vi "Check If Winner Board.vi"(9 "Matriz Status In":bool[][](array[boolean]), 10 "Turn Number":i32, 11 "Boards":i32[][](array[numeric])) -> (1 "Matriz Status Out":bool[][](array[boolean]), 3 "Winner?":bool)   [LabVIEW 2019, in "Day 4.lvlib"]
uses:
  Day 4.lvlib
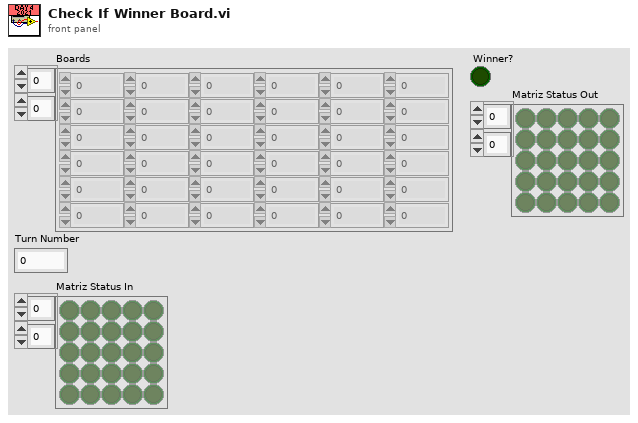
[diagram p1: front panel]
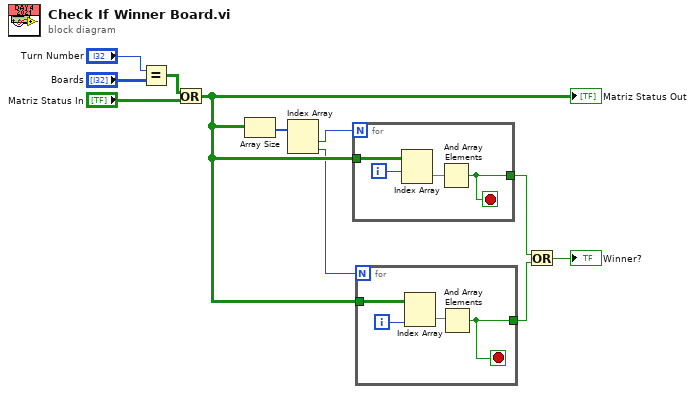
[diagram p0: block diagram]
diagram:
  n1 = Equal?(x="Turn Number", y="Boards") -> (x = y?=w9:bool[][])
  n2 = Or(x=w9, y="Matriz Status In") -> (x .or. y?=w5:bool[][])
  "Matriz Status Out" <- w5
  n3 = Array Size(array=w5) -> (size(s)=w7:i32[])
  n4 = Index Array(array=w7) -> (element #1=w6:i32, element #2=w4:i32)  [unwired: 2 in]
  n5 = for {
    N: w6 -> [_]
    tunnel: w5 -> [w15]
    tunnel: [w12] -> w3
    i -> [w14]
    stop <- w12 stop-if-true
    n6 = Index Array(array=w15, index (row)=w14) -> (element=w13:bool[])  [unwired: 1 in]
    n7 = And Array Elements(Boolean array=w13) -> (logical AND=w12:bool)
  }
  n8 = for {
    N: w4 -> [_]
    tunnel: w5 -> [w19]
    tunnel: [w16] -> w2
    i -> [w18]
    stop <- w16 stop-if-true
    n9 = Index Array(array=w19, index (col)=w18) -> (element=w17:bool[])  [unwired: 1 in]
    n10 = And Array Elements(Boolean array=w17) -> (logical AND=w16:bool)
  }
  n11 = Or(x=w3, y=w2) -> (x .or. y?=→"Winner?":bool)
